vi "Test Code - PSW.vi"() -> ()   [LabVIEW 2011]
uses:
  Password/PSW_01.vi
panel:
  out "found":bool
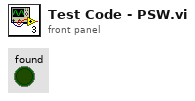
[diagram p1: front panel]
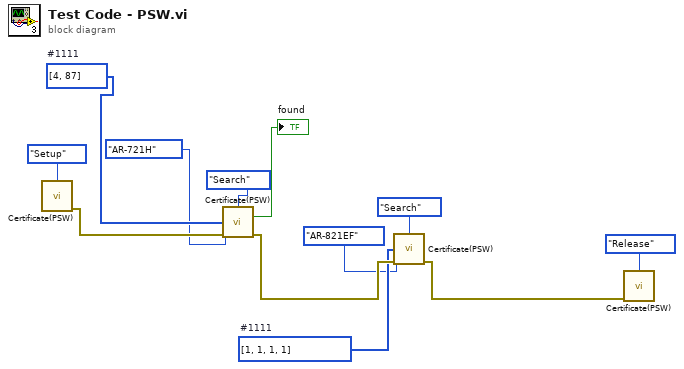
[diagram p0: block diagram]
diagram:
  w8 = u8[] [4, 87]  # #1111
  w3 = u8[] [1, 1, 1, 1]  # #1111
  n1 = call-poly "Certificate(PSW).vi"("select"=enum16{"Setup", "Search", "Release"}."Setup") -> ("error out"=w9:errorcluster)  [unwired: 12 in, 2 out]
  n2 = call-poly "Certificate(PSW).vi"("type"=enum16{"AR-721H", "AR-821EF"}."AR-721H", "select"=enum16{"Setup", "Search", "Release"}."Search", "key"=w8, "error in"=w9) -> ("found"=→"found":bool, "error out"=w5:errorcluster)  [unwired: 9 in, 1 out]
  n3 = call-poly "Certificate(PSW).vi"("type"=enum16{"AR-721H", "AR-821EF"}."AR-821EF", "select"=enum16{"Setup", "Search", "Release"}."Search", "key"=w3, "error in"=w5) -> ("error out"=w4:errorcluster)  [unwired: 9 in, 2 out]
  n4 = call-poly "Certificate(PSW).vi"("select"=enum16{"Setup", "Search", "Release"}."Release", "error in"=w4) -> ()  [unwired: 11 in, 3 out]
